vi "Error Monitor Subpanel.vi"() -> ()   [LabVIEW 2021, in "CIF Manager UI.lvlib"]
uses:
  CIF Manager UI.lvlib
  CIFManagerUI Class/Typedef/Class Data for Manager SubPanel.ctl
  <vilib>/CIF Foundation/CIF Core/CIFUI/Typedef/Class Data for SubPanel.ctl
  <vilib>/CIF Foundation/CIF Core/CIFUI/Typedef/Core UI References.ctl
  <vilib>/CIF Foundation/CIF Core/CIFUI/Typedef/Run Listen Button.ctl
  <vilib>/CIF Foundation/CIF Core/CIFUI/Typedef/SubPanel Events.ctl
  <vilib>/CIF Foundation/CIF Core/CIFUI/Typedef/New Connection Plugin Event Data.ctl
  CIFManagerUI Class/Typedef/Core Manager UI References.ctl
  CIFManagerUI Class/Typedef/Channel Connection.ctl
  CIFManagerUI Class/Typedef/New Plugin.ctl
  CIFManagerUI Class/Typedef/CIF_Manager_UI_Tab.ctl
  CIFPluginManager/typedef/New Connection Event Data.ctl
  <vilib>/gRPC/LabVIEW gRPC Library/Shared/grpcId.ctl
  CIFManagerUI Class/CIF_Manager_UI.lvclass/CIF_Manager_UI.ctl
  <vilib>/CIF Foundation/CIF Core/CIFUI/CIF_UI.lvclass/CIF_UI.ctl
  <vilib>/CIF Foundation/CIF Core/CIFPluginManager/gRPC/CIF_Manager_client/RPC Messages/cif_manager_CreateOrchRequest.ctl
  <vilib>/CIF Foundation/CIF Core/CIFPluginManager/gRPC/CIF_Manager_client/RPC Messages/cif_manager_OrchestrationLanguage.ctl
  <vilib>/CIF Foundation/CIF Core/CIFUI/Utilities/Get Human Readable Error.vi
  <vilib>/CIF Foundation/CIF Utilities/Errors/Append Error Location.vi
  <vilib>/CIF Foundation/CIF Core/CIFUI/Accessors/Read Instrument Studio.vi
  CIFManagerUI Class/CIF_Manager_UI.lvclass
  C:/Program Files/National Instruments/LabVIEW 2021/vi.lib/CIF Foundation/CIF Core/CIFUI/CIF_UI.lvclass
  <vilib>/CIF Foundation/CIF Core/CIFUI/UI Helpers/UI Element Update/Empty Tree by Reference.vi
  CIFManagerUI Class/Manager Functions/SubVIs/Initialize Manager Tab by Reference.vi
  <vilib>/CIF Foundation/CIF Core/CIFUI/UI Helpers/UI Element Update/Empty Table by Reference.vi
  <vilib>/CIF Foundation/CIF Utilities/Errors/Human Readable Error Message.vi
  <vilib>/CIF Foundation/CIF Core/CIFUI/CIF_UI.lvclass
  <vilib>/CIF Foundation/CIF Core/CIFPluginManager/gRPC/CIF_Manager_Client_Wrapper/CIFManagerClientWrapper.lvlib
  <vilib>/CIF Foundation/CIF Core/CIFPluginManager/gRPC/CIF_Manager_client/CIF_Manager_client.lvlib
  <vilib>/CIF Foundation/CIF Core/CIFCore/Grpc/CIFCoreWrapper/CIFCoreWrapper.lvlib
  <vilib>/gRPC/LabVIEW gRPC Library/grpc-lvsupport-release.lvlib
panel:
  in  "Class Data for Manager SubPanel":T1
  in  "Refresh All":bool
  in  "Errors":i32(listbox)=-1
  in  "Reset Errors":bool
  in  "Get All Errors":bool
  in  "Get Config":bool
  in  "Reset Config":bool
  in  "All Config":bool
  out "Config":string
  in  "Generate Orchestration":bool
  in  "File Name":string="orchestrate.py"
  in  "Start Timestamp":u64
  out "Orchestration":string
  in  "Plugin Status":string[][](table)
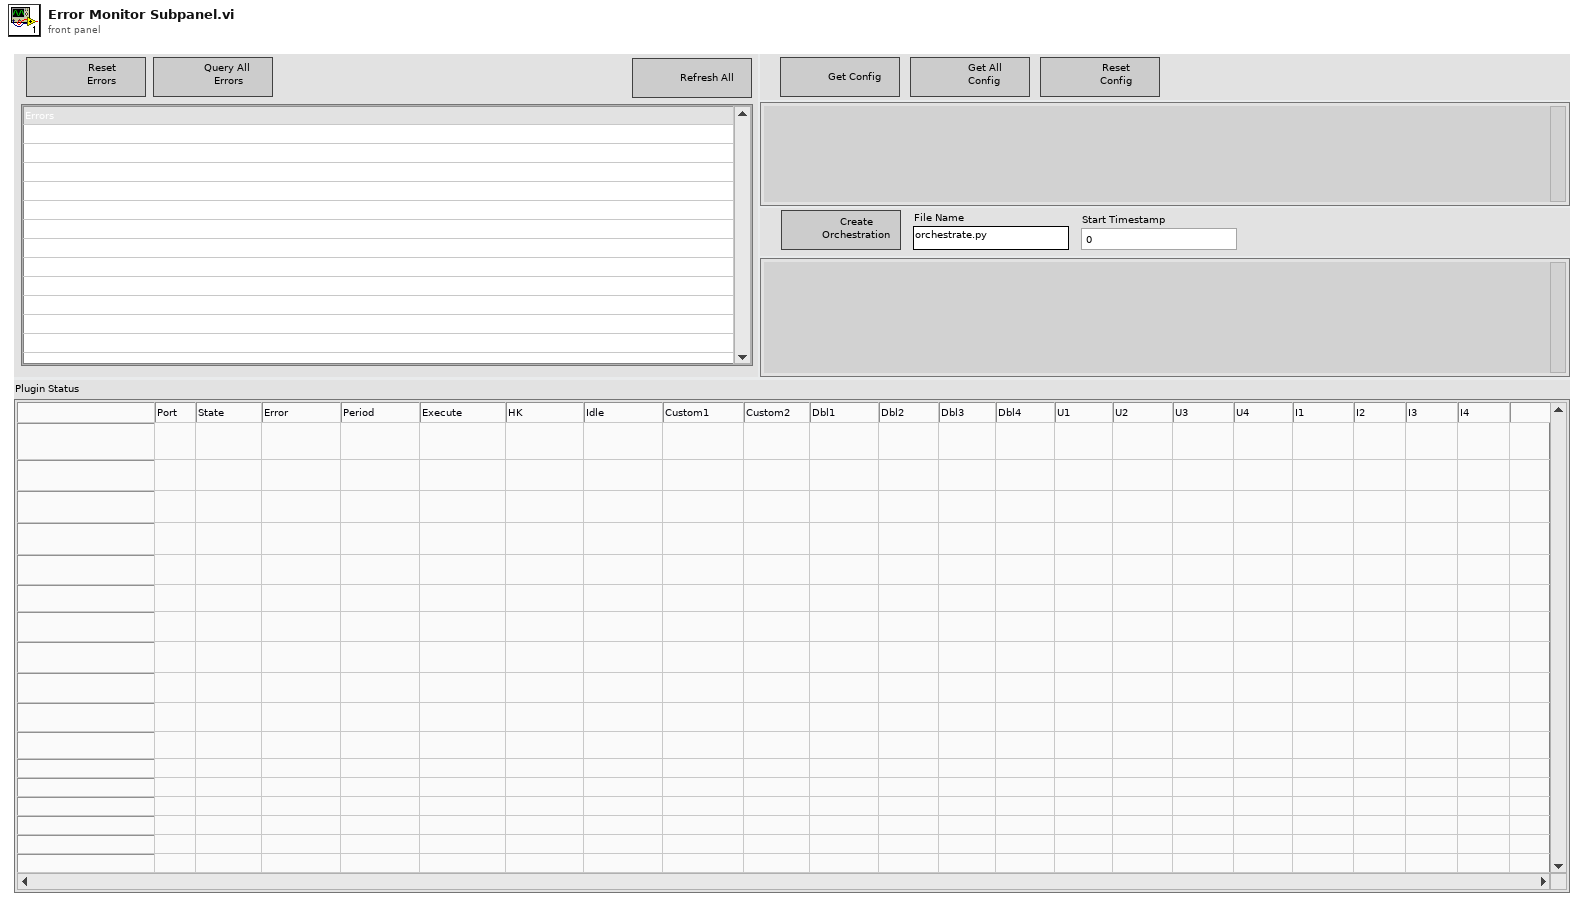
[diagram p1: front panel]
types:
  T1 = typedef "CIF_Manager_UI.lvclass/Class Data for Manager SubPanel.ctl" = cluster{"Class Data for SubPanel":T2, "Manager UI References":T5, "New Manager Connection":refnum<user-event>, "Manager gRPC ID":T6, "Manager Connection":bool}
  T2 = typedef "CIF_UI.lvclass/Class Data for SubPanel.ctl" = cluster{"IP Address":string, "Server Certificate File (.crt)":path, "Connected":bool, "Core UI References":T3, "Subpanel Events":T4, "Manager gRPC Port":i32}
  T3 = typedef "CIF_UI.lvclass/Core UI References.ctl" = cluster{"Plugin Status":refnum<vi>, "Plugin Status Valid":bool, "Connection":refnum<vi>, "Connection Valid":bool, "Exit":refnum<vi>, "Exit Valid":bool, "Run Listen":refnum<vi>, "Run Listen Valid":bool, "Clear Local Error":refnum<vi>, "Clear Local Error Valid":bool, "Local Error":refnum<vi>, "Local Error Valid":bool}
  T4 = typedef "CIF_UI.lvclass/SubPanel Events.ctl" = cluster{"Clear Local Error":refnum<user-event>, "Shutdown":refnum<user-event>, "Plugin Connection":refnum<user-event>}
  T5 = typedef "CIF_Manager_UI.lvclass/Core Manager UI References.ctl" = cluster{"Discovered Plugins":refnum<vi>, "Discovered Plugins Valid":bool, "Loaded Plugins":refnum<vi>, "Loaded Plugins Valid":bool, "Publisher Channels":refnum<vi>, "Publisher Channels Valid":bool, "Subscriber Channels":refnum<vi>, "Subscriber Channels Valid":bool, "Channel Connection":refnum<vi>, "Channel Connection Valid":bool, "New Plugin Load":refnum<vi>, "New Plugin Load Valid":bool, "Errors":refnum<vi>, "Errors Valid":bool, "Plugin to Abort":refnum<vi>, "Plugin to Abort Valid":bool, "CIF Manager Tab":refnum<vi>, "Manger Tab Valid":bool, "System Errors":refnum<vi>, "System Errors Valid":bool, "Plugin Selection":refnum<vi>, "Plugin Selection Valid":bool}
  T6 = typedef "grpc-lvsupport-release.lvlib/grpcId.ctl" = u64
  T7 = typedef "CIF_Manager_client.lvlib/cif_manager_CreateOrchRequest.ctl" = cluster{"start_timestamp":u64, "create_file":bool, "orchestration_language":T8, "filename":string, "default_ip":string}
  T8 = typedef "CIF_Manager_client.lvlib/cif_manager_OrchestrationLanguage.ctl" = enum32{"ORCHESTRATIONLANGUAGE_UNKNOWN", "ORCHESTRATIONLANGUAGE_PYTHON"}
  T9 = typedef "CIF_UI.lvclass/Plugin Connection Map.ctl" = map{string, T10}
  T10 = typedef "CIF_UI.lvclass/Plugin Connections.ctl" = cluster{"gRPC ID":T6, "Plugin Info":T11}
  T11 = typedef "CIFCoreCommon.lvlib/PluginInfo.ctl" = cluster{"Name":string, "Type":string, "grpc_port":i32, "Version":T12, "Node Status":T13}
  T12 = typedef "CIFCoreCommon.lvlib/Version Simple.ctl" = cluster{"Major":i32, "Minor":i32, "Fix":i32}
  T13 = typedef "CIFCoreCommon.lvlib/gRPC Reported Plugin Status.ctl" = cluster{"State":T14, "Timing Statistics (us)":T15, "FIFO Statistics (us)":T17, "error":T18, "Monitor Doubles":T19, "Monitor U64":T20, "Monitor I64":T21}
  T14 = typedef "CIFCoreCommon.lvlib/Plugin State.ctl" = enum32{"Null", "Creating", "Listening", "Running", "CleaningUp", "Destroying"}
  T15 = typedef "CIFCoreCommon.lvlib/Timing Statistics.ctl" = cluster{"Period":T16, "Wake Error":T16, "Execute":T16, "Housekeep":T16, "Idle":T16, "Cleanup":T16, "Custom 1 (custom units)":T16, "Custom 2 (custom units)":T16}
  T16 = typedef "CIFCoreCommon.lvlib/Timing Stats Base.ctl" = cluster{"Max":i64, "Avg":dbl, "Min":i64}
  T17 = typedef "CIFCoreCommon.lvlib/FIFO Statistics.ctl" = cluster{"From T0":T16, "From Previous Plugin":T16, "Output Error":T16}
  T18 = typedef "CIFCoreCommon.lvlib/Simple Error.ctl" = cluster{"status":bool, "code":i32}
  T19 = typedef "CIFCoreCommon.lvlib/Monitor Doubles.ctl" = cluster{"1":dbl, "2":dbl, "3":dbl, "4":dbl}
  T20 = typedef "CIFCoreCommon.lvlib/Monitor U64.ctl" = cluster{"1":u64, "2":u64, "3":u64, "4":u64}
  T21 = typedef "CIFCoreCommon.lvlib/Monitor I64.ctl" = cluster{"1":i64, "2":i64, "3":i64, "4":i64}
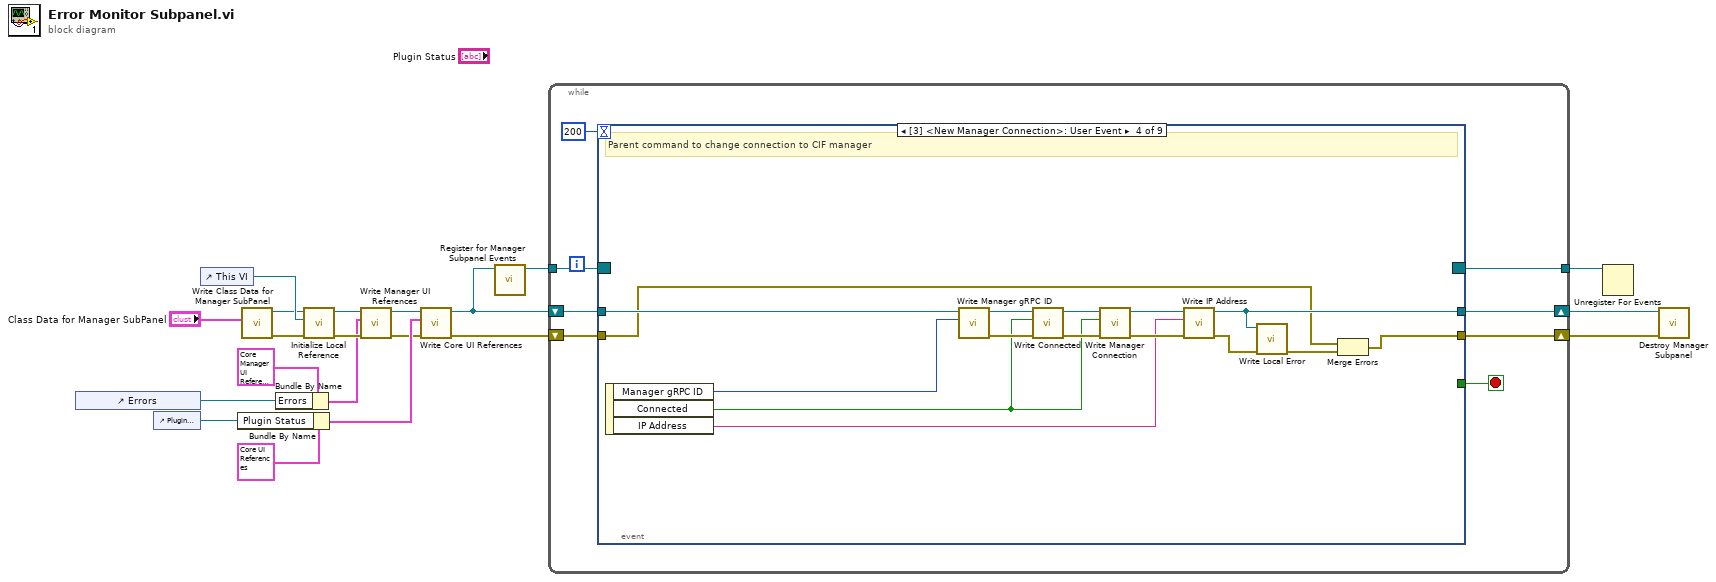
[diagram p0: block diagram]
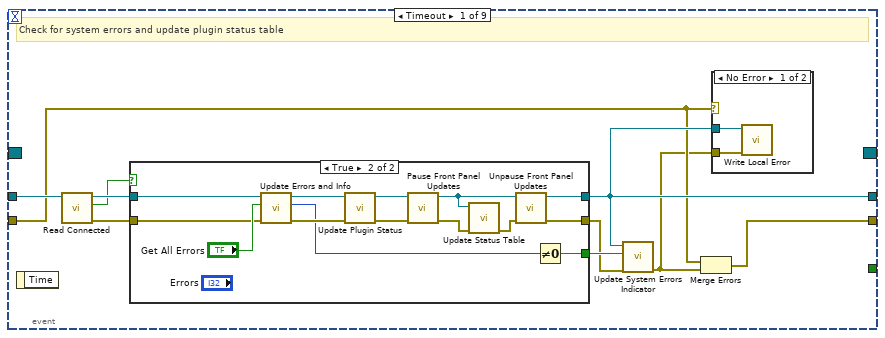
[diagram p2: hidden frame]
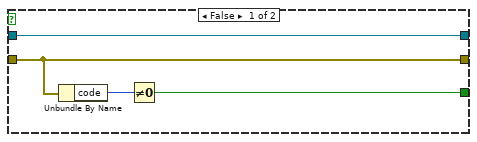
[diagram p4: hidden frame]
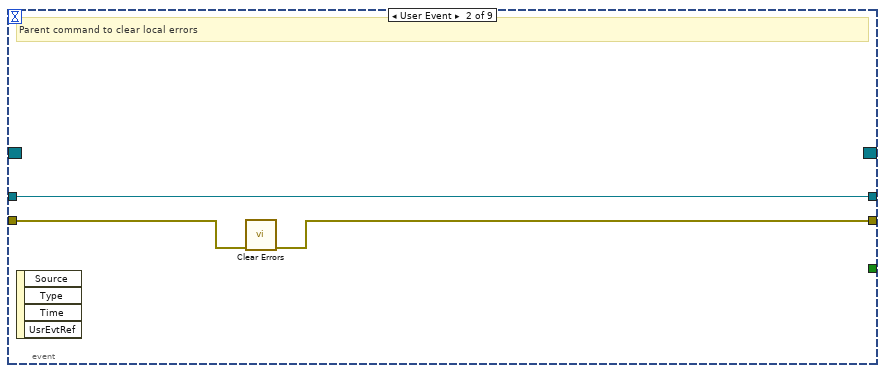
[diagram p5: hidden frame]
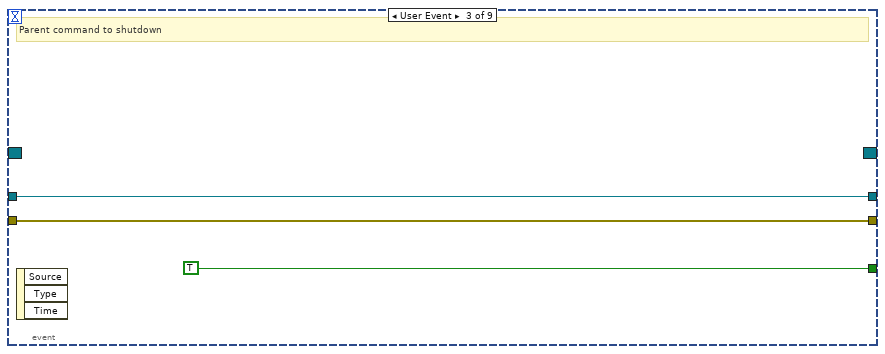
[diagram p6: hidden frame]
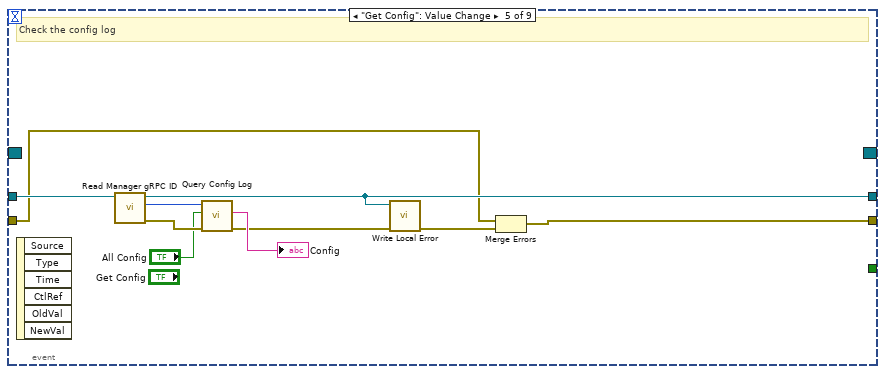
[diagram p7: hidden frame]
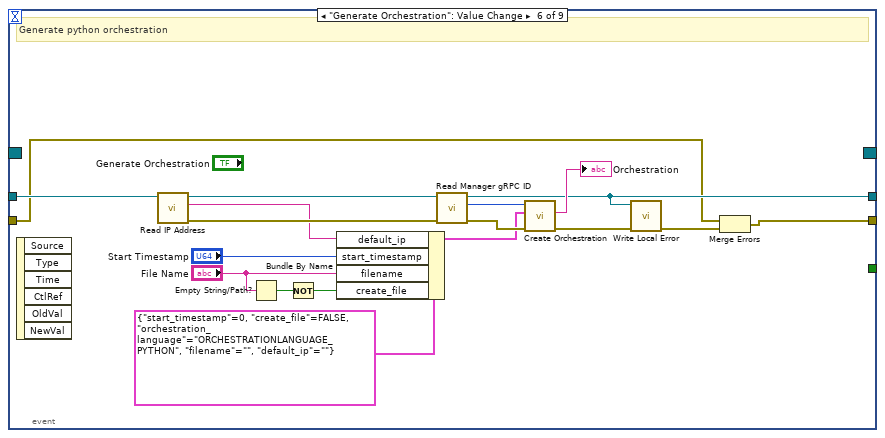
[diagram p8: hidden frame]
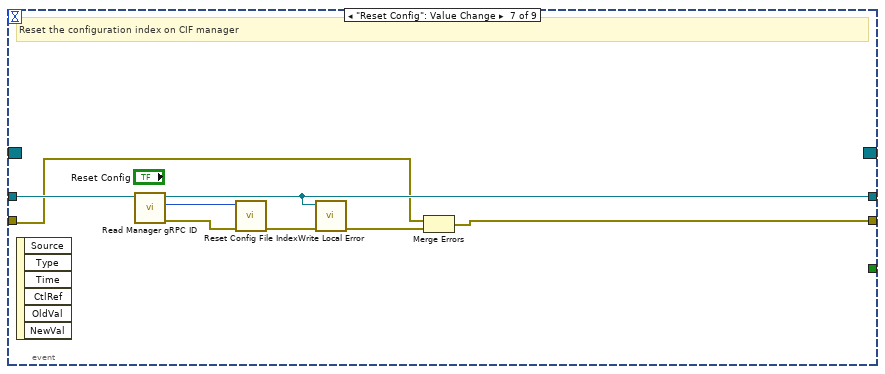
[diagram p9: hidden frame]
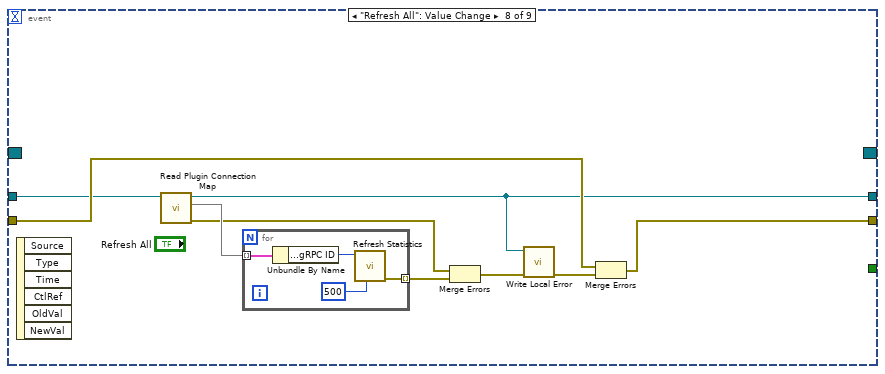
[diagram p10: hidden frame]
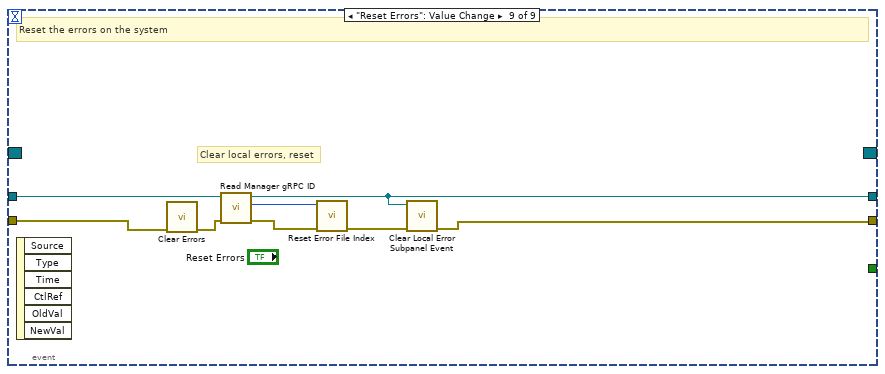
[diagram p11: hidden frame]
diagram:
  n1 = control-ref of="Errors"() -> (w10:refnum<vi>)
  n2 = control-ref of="Plugin Status"() -> (w17:refnum<vi>)
  n3 = control-ref of="This VI"() -> (w16:refnum<vi>)
  n4 = Bundle By Name(cluster=T3 {"Plugin Status"=refnum, "Plugin Status Valid"=FALSE, "Connection"=refnum, "Connection Valid"=FALSE, "Exit"=refnum, "Exit Valid"=FALSE, "Run Listen"=refnum, "Run Listen Valid"=FALSE, "Clear Local Error"=refnum, "Clear Local Error Valid"=FALSE, "Local Error"=refnum, "Local Error Valid"=FALSE} ("UI References"), "Plugin Status"=w17) -> (w18:T3)
  n5 = call "Write Class Data for Manager SubPanel.vi"("Class Data for Manager SubPanel"="Class Data for Manager SubPanel") -> ("error out"=w6:errorcluster, "CIF_Manager_UI out"=w7:refnum<class "CIF_Manager_UI.lvclass">)  [unwired: 9 in]
  n6 = Bundle By Name(cluster=T5 {"Discovered Plugins"=refnum, "Discovered Plugins Valid"=FALSE, "Loaded Plugins"=refnum, "Loaded Plugins Valid"=FALSE, "Publisher Channels"=refnum, "Publisher Channels Valid"=FALSE, "Subscriber Channels"=refnum, "Subscriber Channels Valid"=FALSE, "Channel Connection"=refnum, "Channel Connection Valid"=FALSE, "New Plugin Load"=refnum, "New Plugin Load Valid"=FALSE, "Errors"=refnum, "Errors Valid"=FALSE, "Plugin to Abort"=refnum, "Plugin to Abort Valid"=FALSE, "CIF Manager Tab"=refnum, "Manger Tab Valid"=FALSE, "System Errors"=refnum, "System Errors Valid"=FALSE, "Plugin Selection"=refnum, "Plugin Selection Valid"=FALSE} ("Manager UI References"), "Errors"=w10) -> (w9:T5)
  n7 = call <vilib>:"Initialize Local Reference.vi"("error in (no error)"=w6, "This VI"=w16, "CIF_UI in"=w7) -> ("error out"=w13:errorcluster, "CIF_UI out"=w14:refnum<class "CIF_Manager_UI.lvclass">)  [unwired: 7 in]
  n8 = call "Write Manager UI References.vi"("error in (no error)"=w13, "Manager UI References"=w9, "CIF_UI in"=w14) -> ("error out"=w11:errorcluster, "CIF_UI out"=w12:refnum<class "CIF_Manager_UI.lvclass">)  [unwired: 7 in]
  n9 = call <vilib>:"Write Core UI References.vi"("error in (no error)"=w11, "UI References"=w18, "CIF_UI in"=w12) -> ("error out"=w19:errorcluster, "CIF_UI out"=w4:refnum<class "CIF_Manager_UI.lvclass">)  [unwired: 7 in]
  n10 = call "Register for Manager Subpanel Events.vi"("CIF_Manager_UI in"=w4) -> ("Event Registration Refnum"=w3:refnum<event-registration>)  [unwired: 9 in, 1 out]
  n11 = while {
    shift-right: [w24] -> w1
    shift-left: w4 -> [w26]
    shift-right: [w21] -> w2
    shift-left: w19 -> [w25]
    tunnel: w3 -> [w23]
    tunnel: [w22] -> w15
    stop <- w27 stop-if-true
    n12 = event shown="[3] <New Manager Connection>: User Event" {
      selector: w23 -> [_ _ _ _ _ _ _ _ _]
      dyn-events: [_ _ _ _ _ _ _ _ _] -> w22
      timeout: 200 -> [_ _ _ _ _ _ _ _ _]
      tunnel: [_ _ TRUE _ _ _ _ _ _] -> w27
      tunnel: w26 -> [w35 w59 w63 w73 w85 w104 w113 w122 w134]
      tunnel: w25 -> [w31 w61 w62 w66 w81 w91 w108 w123 w133]
      tunnel: [w29 w60 w62 w65 w80 w92 w109 w117 w129] -> w21
      tunnel: [w32 w59 w63 w68 w84 w95 w112 w116 w130] -> w24
      event Timeout {
        # "Check for system errors and update plugin status table"
        n13 = event-data() -> ()  [unwired: 1 in, 1 out]
        n14 = call <vilib>:"Read Connected.vi"("CIF_UI in"=w35) -> ("error out"=w37:errorcluster, "Connected"=w36:bool, "CIF_UI out"=w38:refnum<class "CIF_Manager_UI.lvclass">)  [unwired: 8 in]
        n15 = case shown="True" w36 {
          tunnel: w37 -> [w43 w53]
          tunnel: [w43 w56] -> w33
          tunnel: w38 -> [w44 w54]
          tunnel: [w44 w55] -> w32
          tunnel: [w41 w58] -> w34
          frame False {
            n16 = Unbundle By Name(w43) -> ("code"=w42:i32)
            n17 = Not Equal To 0?(x=w42) -> (x != 0?=w41:bool)
          }
          frame True {
            n18 = call "Update Errors and Info.vi"("error in (no error)"=w53, "Get All Errors"="Get All Errors", "CIF_UI in"=w54) -> ("error out"=w47:errorcluster, "Error Count"=w45:i32, "CIF_UI out"=w46:refnum<class "CIF_Manager_UI.lvclass">)  [unwired: 5 in, 1 out]
            n19 = call <vilib>:"Update Plugin Status.vi"("error in (no error)"=w47, "CIF_UI in"=w46) -> ("error out"=w50:errorcluster, "CIF_UI out"=w52:refnum<class "CIF_Manager_UI.lvclass">)  [unwired: 8 in]
            n20 = call <vilib>:"Pause Front Panel Updates.vi"("error in (no error)"=w50, "CIF_UI in"=w52) -> ("error out"=w51:errorcluster, "CIF_UI out"=w49:refnum<class "CIF_Manager_UI.lvclass">)  [unwired: 8 in]
            n21 = call <vilib>:"Update Status Table.vi"("error in (no error)"=w51, "CIFManager_UI in"=w49) -> ("error out"=w48:errorcluster)  [unwired: 9 in]
            n22 = call <vilib>:"Unpause Front Panel Updates.vi"("error in (no error)"=w48, "CIF_UI in"=w49) -> ("error out"=w56:errorcluster, "CIF_UI out"=w55:refnum<class "CIF_Manager_UI.lvclass">)  [unwired: 8 in]
            n23 = Not Equal To 0?(x=w45) -> (x != 0?=w58:bool)
          }
        }
        n24 = call "Update System Errors Indicator.vi"("error in (no error)"=w33, "System Errors"=w34, "CIF_UI in"=w32) -> ("error out"=w30:errorcluster)  [unwired: 8 in]
        n25 = Merge Errors(w31, w30) -> (w29:errorcluster)
        n26 = case shown="No Error" w31 {
          tunnel: w32 -> [w40 _]
          tunnel: w30 -> [w39 _]
          frame No Error {
            n27 = call <vilib>:"Write Local Error.vi"("error in (no error)"=w39, "CIF_UI in"=w40) -> ()  [unwired: 9 in, 1 out]
          }
          frame Error {
          }
        }
      }
      event User Event {
        # "Parent command to clear local errors"
        n28 = event-data() -> ()  [unwired: 1 in, 4 out]
        n29 = call <vilib>:"Clear Errors.vi"("error in (no error)"=w61) -> ("error out"=w60:errorcluster)  [unwired: 5 in, 1 out]
      }
      event User Event {
        # "Parent command to shutdown"
        n30 = event-data() -> ()  [unwired: 1 in, 3 out]
      }
      event User Event {
        # "Parent command to change connection to CIF manager"
        n31 = event-data() -> ("Manager gRPC ID"=w70:T6, "Connected"=w71:bool, "IP Address"=w72:string)  [unwired: 1 in]
        n32 = call <vilib>:"Write Manager gRPC ID.vi"("gRPCid"=w70, "CIF_UI in"=w73) -> ("error out"=w78:errorcluster, "CIF_UI out"=w79:refnum<class "CIF_Manager_UI.lvclass">)  [unwired: 8 in]
        n33 = call <vilib>:"Write Connected.vi"("error in (no error)"=w78, "Connected"=w71, "CIF_UI in"=w79) -> ("error out"=w76:errorcluster, "CIF_UI out"=w77:refnum<class "CIF_Manager_UI.lvclass">)  [unwired: 7 in]
        n34 = call <vilib>:"Write Manager Connection.vi"("error in (no error)"=w76, "Manager Connection"=w71, "CIF_UI in"=w77) -> ("error out"=w74:errorcluster, "CIF_UI out"=w75:refnum<class "CIF_Manager_UI.lvclass">)  [unwired: 7 in]
        n35 = call <vilib>:"Write IP Address.vi"("error in (no error)"=w74, "IP Address"=w72, "CIF_UI in"=w75) -> ("error out"=w69:errorcluster, "CIF_UI out"=w68:refnum<class "CIF_Manager_UI.lvclass">)  [unwired: 7 in]
        n36 = call <vilib>:"Write Local Error.vi"("error in (no error)"=w69, "CIF_UI in"=w68) -> ("error out"=w67:errorcluster)  [unwired: 9 in]
        n37 = Merge Errors(w66, w67) -> (w65:errorcluster)
      }
      event "Get Config": Value Change {
        # "Check the config log"
        n38 = event-data() -> ()  [unwired: 1 in, 6 out]
        n39 = call <vilib>:"Read Manager gRPC ID.vi"("CIF_UI in"=w85) -> ("error out"=w88:errorcluster, "Manager gRPCid"=w89:T6, "CIF_UI out"=w84:refnum<class "CIF_Manager_UI.lvclass">)  [unwired: 8 in]
        n40 = call <vilib>:"Query Config Log.vi"("error in"=w88, "query_all"="All Config", "gRPC ID in"=w89) -> ("error out"=w83:errorcluster, "Config"=→"Config":string)  [unwired: 6 in, 1 out]
        n41 = call <vilib>:"Write Local Error.vi"("error in (no error)"=w83, "CIF_UI in"=w84) -> ("error out"=w82:errorcluster)  [unwired: 9 in]
        n42 = Merge Errors(w81, w82) -> (w80:errorcluster)
      }
      event "Generate Orchestration": Value Change {
        # "Generate python orchestration"
        n43 = event-data() -> ()  [unwired: 1 in, 6 out]
        n44 = call <vilib>:"Read IP Address.vi"("CIF_UI in"=w104) -> ("error out"=w102:errorcluster, "IP address"=w100:string, "CIF_UI out"=w103:refnum<class "CIF_Manager_UI.lvclass">)  [unwired: 8 in]
        n45 = Empty String/Path?(string/path="File Name") -> (empty?=w98:bool)
        n46 = Not(x=w98) -> (.not. x?=w97:bool)
        n47 = Bundle By Name(cluster=T7 {"start_timestamp"=0, "create_file"=FALSE, "orchestration_language"=enum."ORCHESTRATIONLANGUAGE_PYTHON", "filename"="", "default_ip"=""} ("Orchestration Config"), "default_ip"=w100, "start_timestamp"="Start Timestamp", "filename"="File Name", "create_file"=w97) -> (w101:T7)
        n48 = call <vilib>:"Read Manager gRPC ID.vi"("error in (no error)"=w102, "CIF_UI in"=w103) -> ("error out"=w105:errorcluster, "Manager gRPCid"=w107:T6, "CIF_UI out"=w95:refnum<class "CIF_Manager_UI.lvclass">)  [unwired: 7 in]
        n49 = call <vilib>:"Create Orchestration.vi"("error in"=w105, "Orchestration Config"=w101, "gRPC ID in"=w107) -> ("error out"=w94:errorcluster, "Orchestration Script"=→"Orchestration":string)  [unwired: 6 in, 1 out]
        n50 = call <vilib>:"Write Local Error.vi"("error in (no error)"=w94, "CIF_UI in"=w95) -> ("error out"=w93:errorcluster)  [unwired: 9 in]
        n51 = Merge Errors(w91, w93) -> (w92:errorcluster)
      }
      event "Reset Config": Value Change {
        # "Reset the configuration index on CIF manager"
        n52 = event-data() -> ()  [unwired: 1 in, 6 out]
        n53 = call <vilib>:"Read Manager gRPC ID.vi"("CIF_UI in"=w113) -> ("error out"=w114:errorcluster, "Manager gRPCid"=w115:T6, "CIF_UI out"=w112:refnum<class "CIF_Manager_UI.lvclass">)  [unwired: 8 in]
        n54 = call <vilib>:"Reset Config File Index.vi"("error in"=w114, "gRPC ID in"=w115) -> ("error out"=w111:errorcluster)  [unwired: 8 in, 1 out]
        n55 = call <vilib>:"Write Local Error.vi"("error in (no error)"=w111, "CIF_UI in"=w112) -> ("error out"=w110:errorcluster)  [unwired: 9 in]
        n56 = Merge Errors(w108, w110) -> (w109:errorcluster)
      }
      event "Refresh All": Value Change {
        n57 = event-data() -> ()  [unwired: 1 in, 6 out]
        n58 = call <vilib>:"Read Plugin Connection Map.vi"("CIF_UI in"=w122) -> ("error out"=w120:errorcluster, "Plugin Connection Map"=w121:T9, "CIF_UI out"=w116:refnum<class "CIF_Manager_UI.lvclass">)  [unwired: 8 in]
        n59 = for {
          tunnel: w121 -> [w128] mode=indexing
          tunnel: [w126] -> w119 mode=indexing
          n60 = Unbundle By Name(w128) -> ("Plugin Connections.gRPC ID"=w127:T6)
          n61 = call <vilib>:"Refresh Statistics.vi"("timeout (ms)"=500, "gRPC ID"=w127) -> ("error out"=w126:errorcluster)  [unwired: 8 in, 1 out]
        }
        n62 = Merge Errors(w120, w119) -> (w118:errorcluster)
        n63 = call <vilib>:"Write Local Error.vi"("error in (no error)"=w118, "CIF_UI in"=w116) -> ("error out"=w124:errorcluster)  [unwired: 9 in]
        n64 = Merge Errors(w123, w124) -> (w117:errorcluster)
      }
      event "Reset Errors": Value Change {
        # "Clear local errors, reset"
        # "Reset the errors on the system"
        n65 = event-data() -> ()  [unwired: 1 in, 6 out]
        n66 = call <vilib>:"Clear Errors.vi"("error in (no error)"=w133) -> ("error out"=w132:errorcluster)  [unwired: 5 in, 1 out]
        n67 = call <vilib>:"Read Manager gRPC ID.vi"("error in (no error)"=w132, "CIF_UI in"=w134) -> ("error out"=w135:errorcluster, "Manager gRPCid"=w136:T6, "CIF_UI out"=w130:refnum<class "CIF_Manager_UI.lvclass">)  [unwired: 7 in]
        n68 = call <vilib>:"Reset Error File Index.vi"("error in"=w135, "gRPC ID in"=w136) -> ("error out"=w131:errorcluster)  [unwired: 8 in, 1 out]
        n69 = call <vilib>:"Clear Local Error Subpanel Event.vi"("error in (no error)"=w131, "CIF_UI in"=w130) -> ("error out"=w129:errorcluster)  [unwired: 9 in]
      }
    }
  }
  n70 = Unregister For Events(event registration refnum=w15) -> ()  [unwired: 1 in, 1 out]
  n71 = call "Destroy Manager Subpanel.vi"("error in (no error)"=w2, "CIF_Manager_UI in"=w1) -> ()  [unwired: 8 in, 2 out]
